vi "Move.vi"(8 "Error In":errorcluster, 11 "Position":T1(ring)) -> (0 "Error Out":errorcluster)   [LabVIEW 2019, in "IDEX.lvlib"]
uses:
  IDEX.lvlib
  Queues/Queues.lvlib
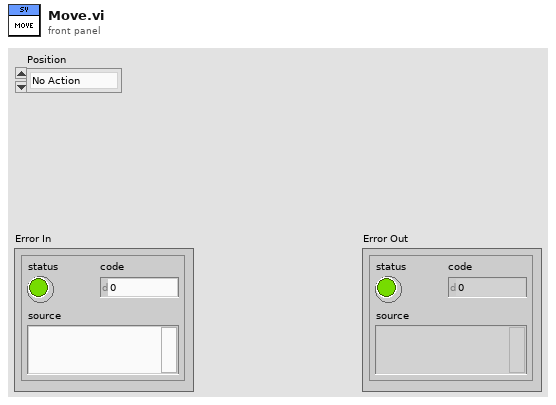
[diagram p1: front panel]
types:
  T1 = enum16{"No Action", "Position 1", "Position 2", "Position 3", "Position 4", "Position 5", "Position 6"}
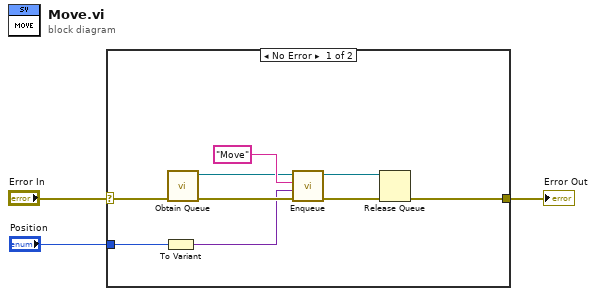
[diagram p0: block diagram]
diagram:
  n1 = case shown="No Error" "Error In" {
    selector: "Error In" -> [w8 w13]
    tunnel: [w9 w13] -> w3
    tunnel: "Position" -> [w5 _]
    frame No Error {
      n2 = To Variant(anything=w5) -> (Variant=w4:variant)
      n3 = call "Obtain Queue.vi"("Error In"=w8) -> ("Error Out"=w7:errorcluster, "Queue out"=w6:refnum<queue>)  [unwired: 9 in]
      n4 = call "Enqueue.vi"("Error In"=w7, "Data"=w4, "State"="Move", "Queue in"=w6) -> ("Error Out"=w11:errorcluster, "Queue out"=w10:refnum<queue>)  [unwired: 6 in]
      n5 = Release Queue(queue=w10, error in (no error)=w11) -> (error out=w9:errorcluster)  [unwired: 1 in, 2 out]
    }
    frame Error {
    }
  }
  "Error Out" <- w3
